vi "Elapsed Time.vi"(8 "seconds since 1Jan1904":timestamp, 9 "Time Target (s)":dbl=177.0) -> (2 "Elapsed Time End":bool, 3 "Time Remaining":dbl)   [LabVIEW 2013]
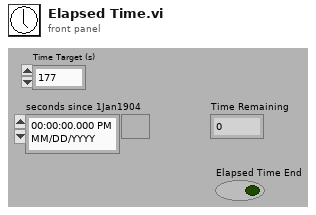
[diagram p1: front panel]
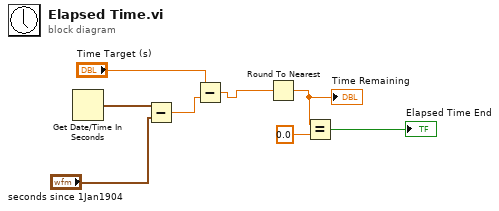
[diagram p0: block diagram]
diagram:
  n1 = Get Date/Time In Seconds() -> (seconds since 1Jan1904=w4:timestamp)
  n2 = Subtract(x=w4, y="seconds since 1Jan1904") -> (x-y=w6:dbl)
  n3 = Subtract(x="Time Target (s)", y=w6) -> (x-y=w2:dbl)
  n4 = Round To Nearest(number=w2) -> (nearest integer value=w1:dbl)
  "Time Remaining" <- w1
  n5 = Equal?(x=w1, y=0.0) -> (x = y?=→"Elapsed Time End":bool)
